vi "Build Settings Box Text.vi"(7 "error in (no error)":errorcluster, 9 "Path to XML":path, 10 "Scan Setup":T1) -> (0 "error out":errorcluster, 3 "settings box text":string)   [LabVIEW 2017, in "Scan Driver.lvclass"]
uses:
  Scan Driver.lvclass
  Scan Setup Mode.ctl
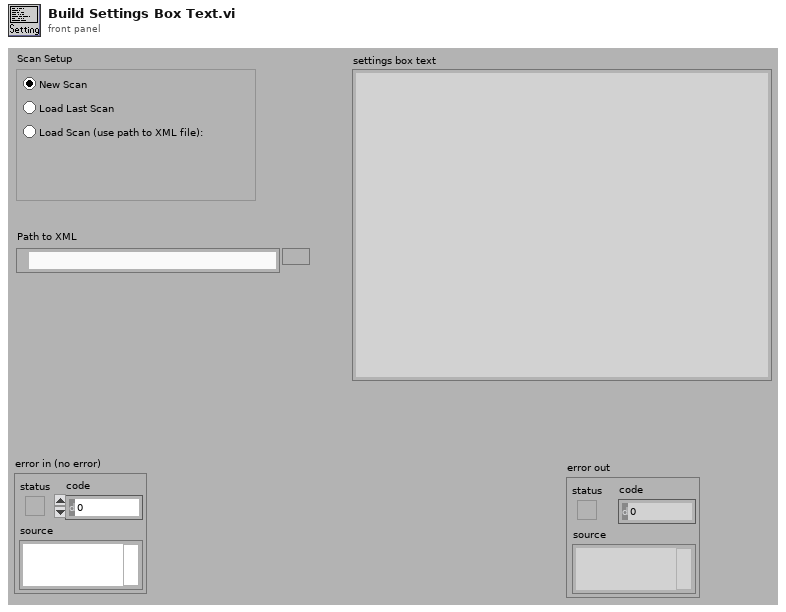
[diagram p1: front panel]
types:
  T1 = typedef "Scan Driver.lvclass/Scan Setup Mode.ctl" = enum32{"New Scan", "Load Last Scan", "Load Scan:"}
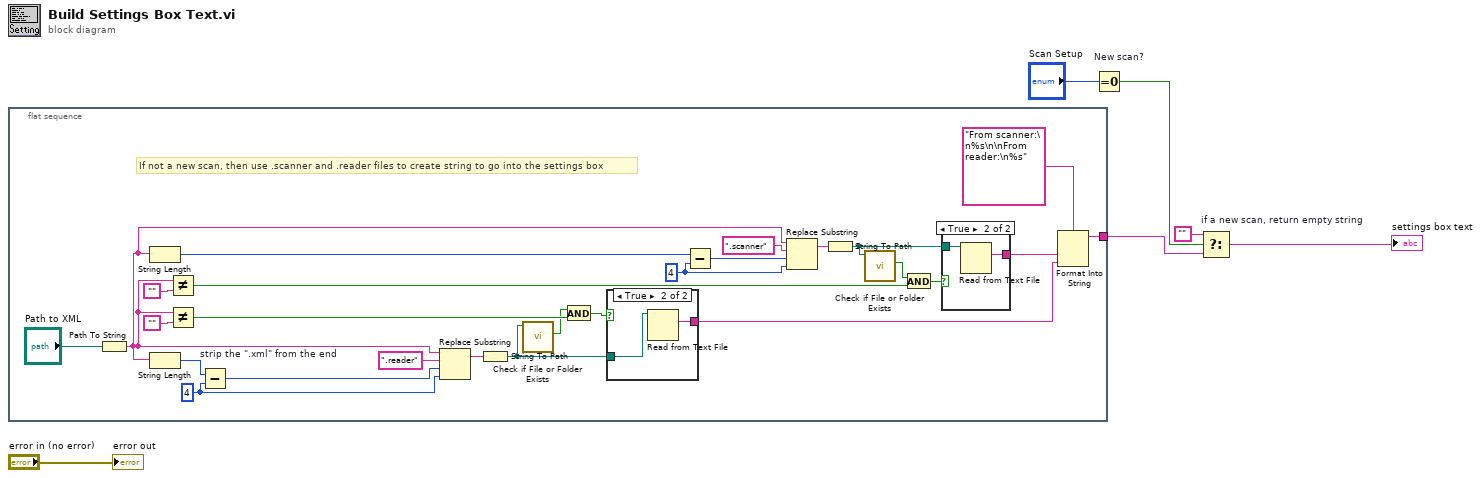
[diagram p0: block diagram]
diagram:
  n1 = flat-sequence {
    tunnel: [w7] -> w4
    frame #0 {
      w20 = 4
      w15 = 4
      # "If not a new scan, then use .scanner and .reader files to create string to go into the settings box"
      n2 = Path To String(path="Path to XML") -> (string=w31:string)
      n3 = String Length(string=w31) -> (length=w13:i32)
      n4 = String Length(string=w31) -> (length=w18:i32)
      n5 = Not Equal?(x=w31, y="") -> (x != y?=w32:bool)
      n6 = Not Equal?(x=w31, y="") -> (x != y?=w28:bool)
      n7 = Subtract "strip the \".xml\" from the end"(x=w18, y=w20) -> (x-y=w19:i32)
      n8 = Replace Substring(2:w20, 3:w19, 4:".reader", 5:w31) -> (1:w21:string)  [unwired: 1 out]
      n9 = String To Path(string=w21) -> (path=w24:path)
      n10 = call <vilib>:"Check if File or Folder Exists.vi"("path"=w24) -> ("file or folder exists?"=w25:bool)  [unwired: 8 in, 2 out]
      n11 = And(x=w25, y=w28) -> (x .and. y?=w26:bool)
      n12 = case shown="True" w26 {
        tunnel: w24 -> [_ w34]
        tunnel: [_ w33] -> w8
        frame False {
        }
        frame True {
          n13 = Read from Text File(file (use dialog)=w34) -> (text=w33:string)  [unwired: 3 in, 3 out]
        }
      }
      n14 = Subtract(x=w13, y=w15) -> (x-y=w14:i32)
      n15 = Replace Substring(2:w15, 3:w14, 4:".scanner", 5:w31) -> (1:w16:string)  [unwired: 1 out]
      n16 = String To Path(string=w16) -> (path=w22:path)
      n17 = call <vilib>:"Check if File or Folder Exists.vi"("path"=w22) -> ("file or folder exists?"=w23:bool)  [unwired: 8 in, 2 out]
      n18 = And(x=w23, y=w32) -> (x .and. y?=w29:bool)
      n19 = case shown="True" w29 {
        tunnel: w22 -> [_ w36]
        tunnel: [_ w35] -> w9
        frame False {
        }
        frame True {
          n20 = Read from Text File(file (use dialog)=w36) -> (text=w35:string)  [unwired: 3 in, 3 out]
        }
      }
      n21 = Format Into String(format string="From scanner:\n%s\n\nFrom reader:\n%s", w9, w8) -> (resulting string=w7:string)  [unwired: 2 in, 1 out]
    }
  }
  n22 = Equal To 0? "New scan?"(x="Scan Setup") -> (x = 0?=w3:bool)
  n23 = Select "if a new scan, return empty string"(t="", s=w3, f=w4) -> (s? t:f=→"settings box text":string)
  "error out" <- "error in (no error)"
